vi "报警信息.vi"() -> ()   [LabVIEW 2020]
panel:
  out "报警信息":string[][](table)
  # "报警信息"
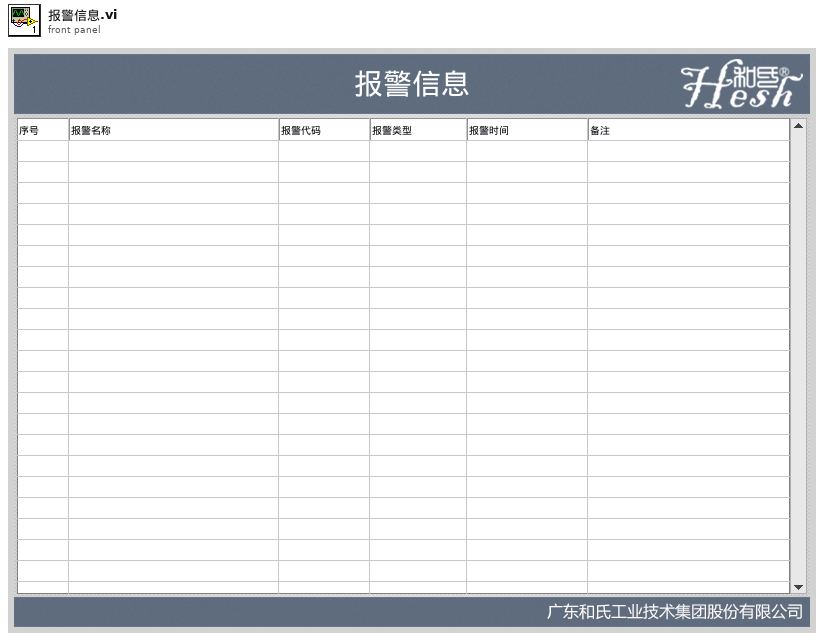
[diagram p1: front panel]
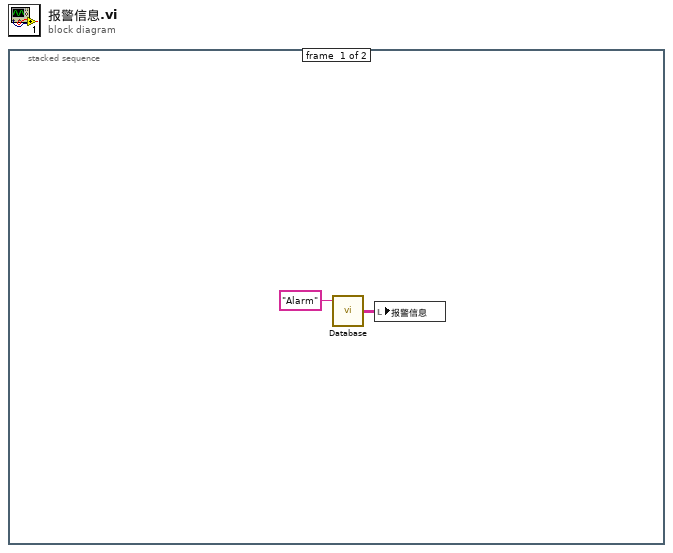
[diagram p0: block diagram]
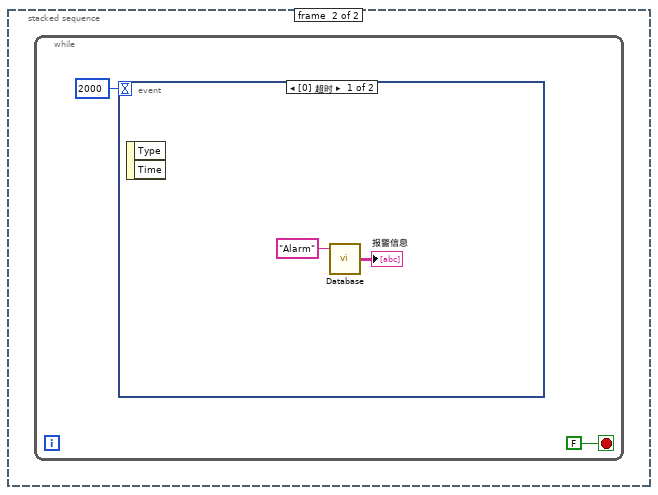
[diagram p2: hidden frame]
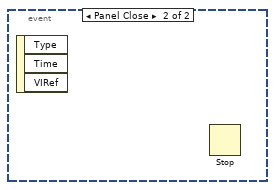
[diagram p3: hidden frame]
diagram:
  n1 = stacked-sequence {
    frame #0 {
      n2 = call "Database.vi"("table"="Alarm") -> ("data"=w2:string[][])  [unwired: 2 in, 2 out]
      n3 = local write "报警信息"(w2) -> ()
    }
    frame #1 {
      n4 = while {
        stop <- FALSE stop-if-true
        n5 = event shown="[0] 超时" {
          selector: _ -> [_ _]
          dyn-events: _ -> [_ _]
          timeout: 2000 -> [_ _]
          event Timeout {
            n6 = event-data() -> ()  [unwired: 1 in, 2 out]
            n7 = call "Database.vi"("table"="Alarm") -> ("data"=→"报警信息":string[][])  [unwired: 2 in, 2 out]
          }
          event Panel Close {
            n8 = event-data() -> ()  [unwired: 1 in, 3 out]
            n9 = Stop() -> ()  [unwired: 1 in]
          }
        }
      }
    }
  }
